vi "SwerveChooseAngle (SubVI).vi"(8 "Hysteresis (deg)":dbl, 9 "Goal Angle (deg)":dbl, 10 "Current Angle (deg)":dbl, 11 "Zero Wheels":bool) -> (0 "Using Hysteresis":bool, 2 "Invert Speed Motor":bool, 3 "Angular Distance":dbl)   [LabVIEW 2020]
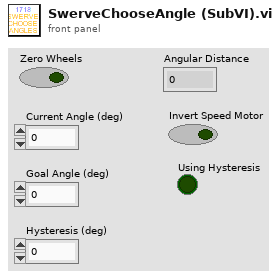
[diagram p1: front panel]
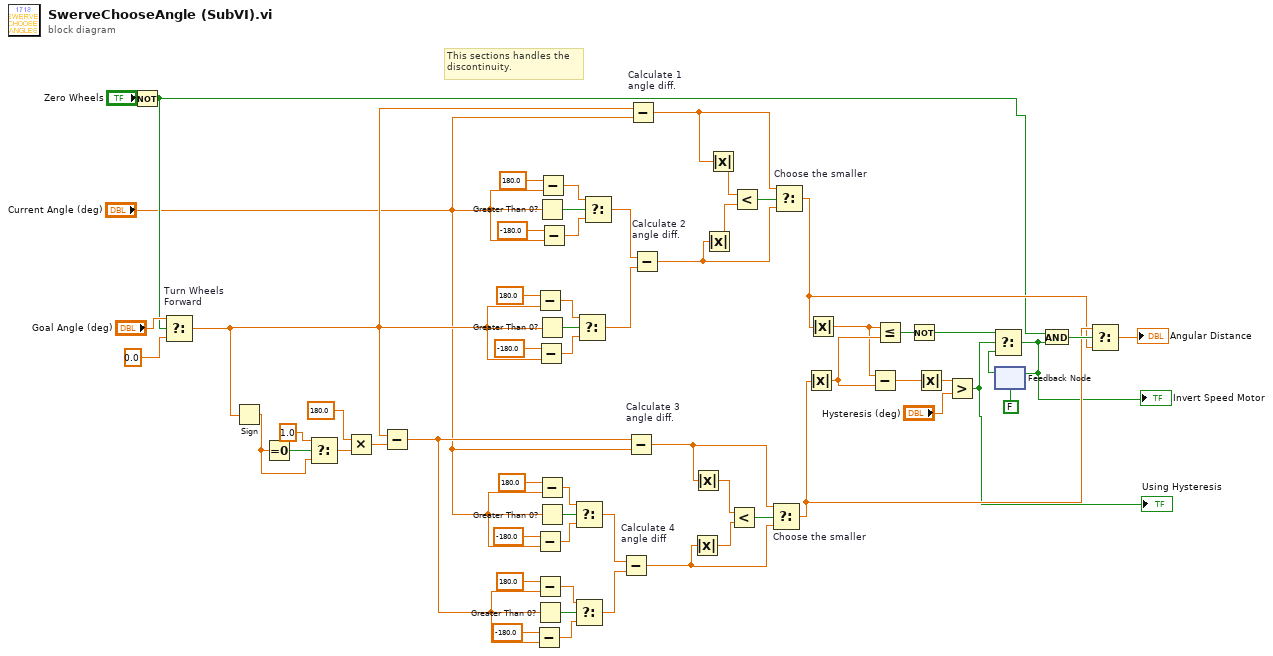
[diagram p0: block diagram]
diagram:
  # "This sections handles the\ndiscontinuity."
  n1 = Not(x="Zero Wheels") -> (.not. x?=w2:bool)
  n2 = Select "Turn Wheels\nForward"(t="Goal Angle (deg)", s=w2, f=0.0) -> (s? t:f=w45:dbl)
  n3 = Sign(1:w45) -> (0:w46:dbl)
  n4 = Equal To 0?(x=w46) -> (x = 0?=w44:bool)
  n5 = Select(t=1.0, s=w44, f=w46) -> (s? t:f=w41:dbl)
  n6 = Multiply(x=180.0, y=w41) -> (x*y=w40:dbl)
  n7 = Subtract(x=w45, y=w40) -> (x-y=w42:dbl)
  n8 = Subtract(x=-180.0, y=w42) -> (x-y=w33:dbl)
  n9 = Subtract(x=180.0, y=w45) -> (x-y=w12:dbl)
  n10 = Subtract(x=-180.0, y="Current Angle (deg)") -> (x-y=w34:dbl)
  n11 = Subtract(x=180.0, y=w42) -> (x-y=w31:dbl)
  n12 = Greater Than 0?(x=w42) -> (x > 0?=w32:bool)
  n13 = Subtract(x=-180.0, y=w45) -> (x-y=w10:dbl)
  n14 = Greater Than 0?(x="Current Angle (deg)") -> (x > 0?=w8:bool)
  n15 = Greater Than 0?(x=w45) -> (x > 0?=w11:bool)
  n16 = Subtract(x=180.0, y="Current Angle (deg)") -> (x-y=w36:dbl)
  n17 = Greater Than 0?(x="Current Angle (deg)") -> (x > 0?=w35:bool)
  n18 = Subtract(x=180.0, y="Current Angle (deg)") -> (x-y=w7:dbl)
  n19 = Subtract(x=-180.0, y="Current Angle (deg)") -> (x-y=w9:dbl)
  n20 = Select(t=w36, s=w35, f=w34) -> (s? t:f=w28:dbl)
  n21 = Select(t=w31, s=w32, f=w33) -> (s? t:f=w27:dbl)
  n22 = Select(t=w12, s=w11, f=w10) -> (s? t:f=w16:dbl)
  n23 = Select(t=w7, s=w8, f=w9) -> (s? t:f=w15:dbl)
  n24 = Subtract "Calculate 4\nangle diff"(x=w28, y=w27) -> (x-y=w22:dbl)
  n25 = Subtract "Calculate 3\nangle diff."(x=w42, y="Current Angle (deg)") -> (x-y=w24:dbl)
  n26 = Subtract "Calculate 1\nangle diff."(x=w45, y="Current Angle (deg)") -> (x-y=w19:dbl)
  n27 = Subtract "Calculate 2\nangle diff."(x=w15, y=w16) -> (x-y=w21:dbl)
  n28 = Absolute Value(x=w22) -> (abs(x)=w25:dbl)
  n29 = Absolute Value(x=w24) -> (abs(x)=w26:dbl)
  n30 = Absolute Value(x=w21) -> (abs(x)=w18:dbl)
  n31 = Absolute Value(x=w19) -> (abs(x)=w17:dbl)
  n32 = Less?(x=w26, y=w25) -> (x < y?=w23:bool)
  n33 = Less?(x=w17, y=w18) -> (x < y?=w20:bool)
  n34 = Select "Choose the smaller"(t=w24, s=w23, f=w22) -> (s? t:f=w59:dbl)
  n35 = Select "Choose the smaller"(t=w19, s=w20, f=w21) -> (s? t:f=w58:dbl)
  n36 = Absolute Value(x=w59) -> (abs(x)=w51:dbl)
  n37 = Absolute Value(x=w58) -> (abs(x)=w50:dbl)
  n38 = Subtract(x=w50, y=w51) -> (x-y=w47:dbl)
  n39 = Less Or Equal?(x=w50, y=w51) -> (x <= y?=w54:bool)
  n40 = Not(x=w54) -> (.not. x?=w55:bool)
  n41 = Absolute Value(x=w47) -> (abs(x)=w48:dbl)
  n42 = Greater?(x=w48, y="Hysteresis (deg)") -> (0:w53:bool)
  "Using Hysteresis" <- w53
  n43 = feedback #1(FALSE) -> (w52:bool)
  n44 = Select(t=w55, s=w53, f=w52) -> (s? t:f=w57:bool)
  "Invert Speed Motor" <- w57
  n45 = feedback-in #1(w57) -> ()
  n46 = And(x=w2, y=w57) -> (x .and. y?=w60:bool)
  n47 = Select(t=w59, s=w60, f=w58) -> (s? t:f=→"Angular Distance":dbl)
